vi "PMX_OpenPMXBrowser.vi"(8 "Error in":errorcluster, 11 "Device":refnum<k24>) -> (0 "Error out":errorcluster, 3 "Device":refnum<k24>)   [LabVIEW 2016]
doc: "Opens the default web browser to show the configuration panel for the given PMX device"
uses:
  <vilib>/Platform/browser.llb/Open URL in Default Browser (string).vi
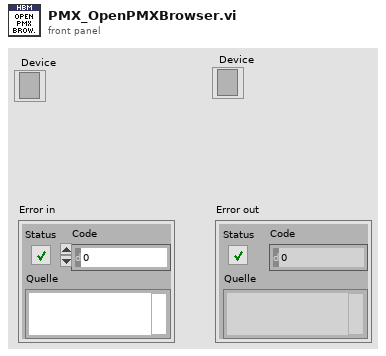
[diagram p1: front panel]
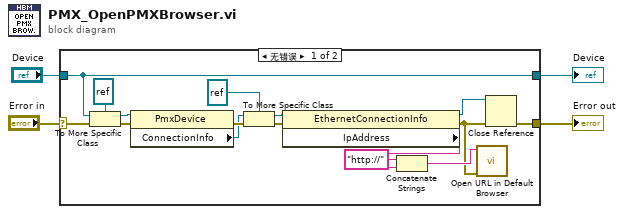
[diagram p0: block diagram]
diagram:
  n1 = case shown="无错误" "Error in" {
    selector: "Error in" -> [w9 w22]
    tunnel: [w5 w22] -> w2
    tunnel: "Device" -> [w10 w21]
    tunnel: [w10 w21] -> w3
    frame No Error {
      n2 = To More Specific Class(target class=refnum<k24> refnum ("Zielklasse"), reference=w10, error in=w9) -> (specific class reference=w20:refnum<k24>, error out=w19:errorcluster)
      n3 = property on="Eigenschaftsknoten" class="PmxDevice"(reference=w20, error in=w19) -> (error out=w18:errorcluster, "ConnectionInfo"=w17:refnum<k24>)  [unwired: 1 out]
      n4 = To More Specific Class(target class=refnum<k24> refnum (".NET (Referenz)"), reference=w17, error in=w18) -> (specific class reference=w16:refnum<k24>, error out=w15:errorcluster)
      n5 = property on="Eigenschaftsknoten" class="EthernetConnectionInfo"(reference=w16, error in=w15) -> (reference out=w6:refnum<k24>, error out=w7:errorcluster, "IpAddress"=w13:string)
      n6 = Concatenate Strings("http://" ("String"), w13) -> (w12:string)
      n7 = call-poly <vilib>:"Open URL in Default Browser.vi"("error in (no error)"=w7, "URL"=w12) -> ()  [unwired: 4 in, 2 out]
      n8 = Close Reference(reference=w6, error in (no error)=w7) -> (error out=w5:errorcluster)
    }
    frame Error {
    }
  }
  "Device" <- w3
  "Error out" <- w2
